vi "Verify Cycle Rounting time.vi"(0 "GEA2 Reference In":refnum<k24>, 5 "ECT Data In":T1, 11 "Error In":errorcluster) -> (4 "GEA2 Reference Out":refnum<k24>, 6 "Routing ECT pass/fail":bool, 8 "Report Text Cycle Routing":string, 15 "Error Out":errorcluster)   [LabVIEW 2016, in "TLMB.lvlib"]
doc: "This vi can be used to read ERD every 1 sec for user selected repeat counts."
uses:
  Projects/TLMB.lvlib
  Q:/Common/DLLs/GEA3/GeaCommunication.dll
  Common/DLLs/GEA3/GeaCommunication.dll
  Controls/ECT.ctl
  Common/LabVIEW GEA2 Toolkit/LabVIEW_GEA2_Toolkit.lvlibp/type defs/Source_Destination.ctl
  Common/LabVIEW GEA2 Toolkit/LabVIEW_GEA2_Toolkit.lvlibp/type defs/ERD Read Data In.ctl
  Common/LabVIEW GEA2 Toolkit/LabVIEW_GEA2_Toolkit.lvlibp/type defs/Data Type.ctl
  Common/LabVIEW GEA2 Toolkit/LabVIEW_GEA2_Toolkit.lvlibp
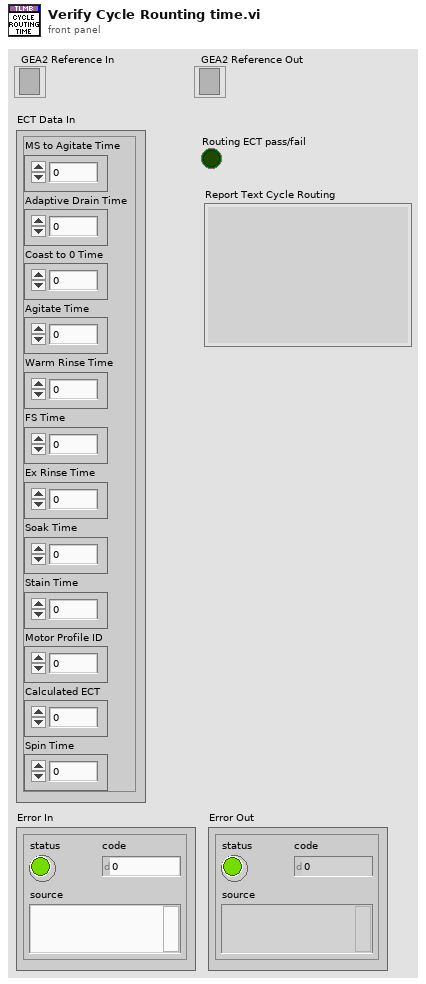
[diagram p1: front panel]
types:
  T1 = typedef "TLMB.lvlib/ECT.ctl" = cluster{"MS to Agitate Time":u16, "Adaptive Drain Time":u16, "Coast to 0 Time":u16, "Agitate Time":u16, "Warm Rinse Time":u16, "FS Time":u16, "Ex Rinse Time":u16, "Soak Time":u16, "Stain Time":u16, "Motor Profile ID":u16, "Calculated ECT":u16, "Spin Time":u16}
  T2 = typedef "LabVIEW_GEA2_Toolkit.lvlibp/Source_Destination.ctl" = cluster{"Source":u8, "Destination":u8}
  T3 = typedef "LabVIEW_GEA2_Toolkit.lvlibp/ERD Read Data In.ctl" = cluster{"ERD Number":u16, "Data Type":T4}
  T4 = typedef "LabVIEW_GEA2_Toolkit.lvlibp/Data Type.ctl" = enum16{"string", "boolean", "uint8_t", "uint16_t", "uint32_t", "uint64_t", "int8_t", "int16_t", "int32_t", "int64_t"}
  T5 = enum16{"EQ (==)", "NE (!=)", "GT (>)", "LT (<)", "GE (>=)", "LE (<=)", "GTLT(> <)", "GELE (>= <=)", "GELT (>= <)", "GTLE (> <=)", "LTGT (< >)", "LEGE (<= >=)", "LEGT (<= >)", "LTGE (< >=)", "No Comparison"}
  T6 = typedef "LabVIEW_GEA2_Toolkit.lvlibp/ERD Read Data Out.ctl" = cluster{"ERD Number":u16, "Data":string}
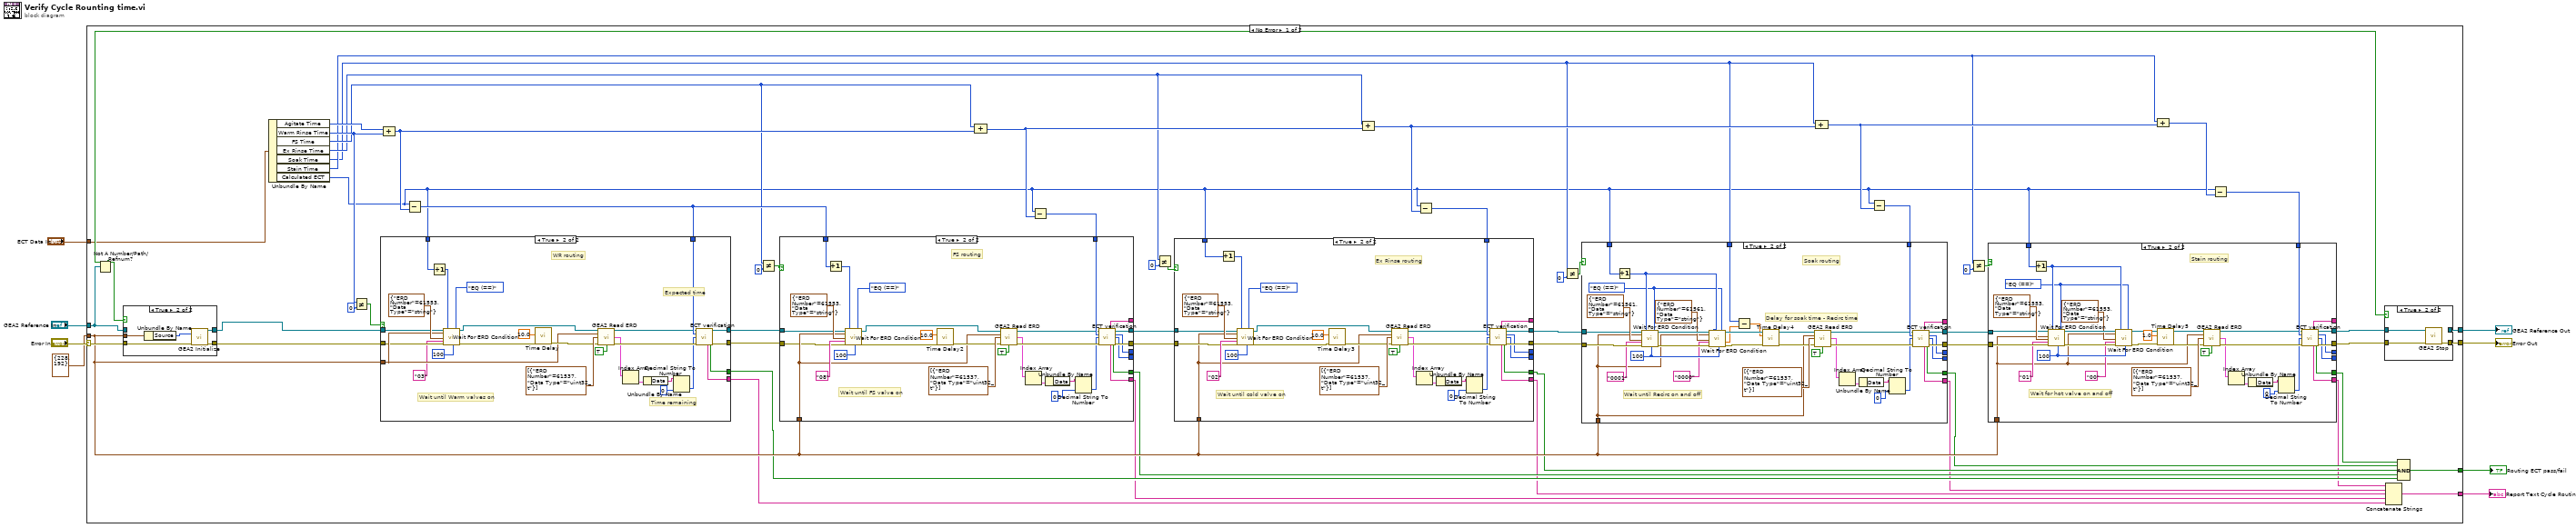
[diagram p0: block diagram]
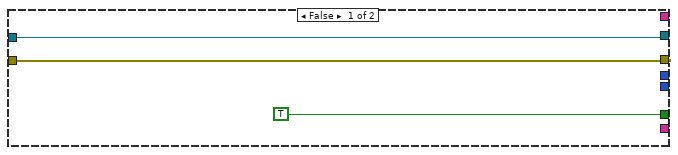
[diagram p2: hidden frame]
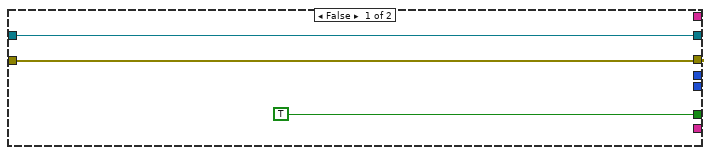
[diagram p3: hidden frame]
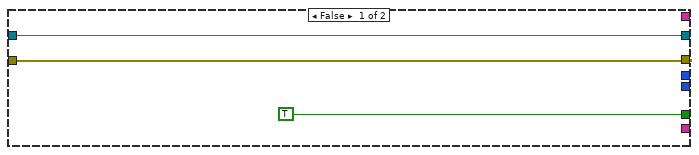
[diagram p4: hidden frame]
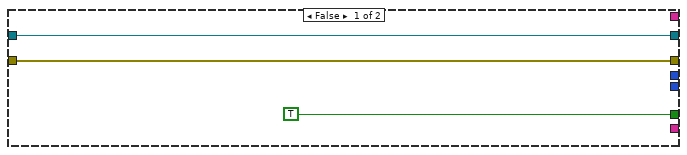
[diagram p5: hidden frame]
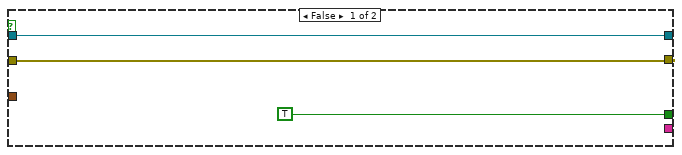
[diagram p6: hidden frame]
diagram:
  n1 = case shown="No Error" "Error In" {
    selector: "Error In" -> [w65 w251]
    tunnel: T2 {"Source"=228, "Destination"=192} ("GEA Inputs") -> [w43 _]
    tunnel: "GEA2 Reference In" -> [w66 w252]
    tunnel: [w62 w252] -> w6
    tunnel: [w64 w251] -> w5
    tunnel: "ECT Data In" -> [w10 _]
    tunnel: [w25 _] -> w3
    tunnel: [w24 _] -> w2
    frame No Error {
      n2 = Not A Number/Path/Refnum?(number/path/refnum=w66) -> (NaN/Path/Refnum?=w63:bool)
      n3 = case shown="True" w63 {
        tunnel: w65 -> [w245 w250]
        tunnel: [w245 w249] -> w9
        tunnel: [w244 w248] -> w12
        tunnel: w43 -> [_ w246]
        tunnel: w66 -> [w244 _]
        frame False {
        }
        frame True {
          n4 = Unbundle By Name(w246) -> ("Source"=w247:u8)
          n5 = call "GEA2 Initialize.vi"("Source Address"=w247, "error in"=w250) -> ("GEA2 Reference Out"=w248:refnum<k24>, "error out"=w249:errorcluster)  [unwired: 11 in, 1 out]
        }
      }
      n6 = Unbundle By Name(w10) -> ("Agitate Time"=w61:u16, "Warm Rinse Time"=w55:u16, "FS Time"=w51:u16, "Ex Rinse Time"=w46:u16, "Soak Time"=w23:u16, "Stain Time"=w36:u16, "Calculated ECT"=w11:u16)
      n7 = Not Equal?(x=w55, y=u16 0) -> (x != y?=w21:bool)
      n8 = Compound Arithmetic op=ADD(w61, w55) -> (w59:u16)
      n9 = Subtract(x=w11, y=w59) -> (x-y=w52:u16)
      n10 = case shown="True" w21 {
        tunnel: [w211 w237] -> w54
        tunnel: [w210 w236] -> w53
        tunnel: w52 -> [_ w230]
        tunnel: [TRUE ("ECT Pass/Fail") w229] -> w35
        tunnel: [_ w228] -> w31
        tunnel: w43 -> [_ w227]
        tunnel: w12 -> [w211 w226]
        tunnel: w9 -> [w210 w225]
        tunnel: w11 -> [_ w215]
        frame False {
        }
        frame True {
          # "Expected time"
          # "Time remaining"
          # "Wait until Warm valves on"
          # "WR routing"
          n11 = Increment(x=w215) -> (x+1=w214:u16)
          n12 = call "Wait For ERD Condition.vi"("GEA2 Reference In"=w226, "GEA Inputs"=w227, "ERD Read Data"=T3 {"ERD Number"=61553, "Data Type"=enum."string"}, "Expected Low"="03", "Error In"=w225, "Timeout (s)"=w214, "Loop Rate (ms)"=u32 100, "Comparison"=T5."EQ (==)") -> ("GEA2 Reference Out"=w217:refnum<k24>, "Error Out"=w216:errorcluster)  [unwired: 7 in, 3 out]
          n13 = call "Time Delay"("error in (no error)"=w216, "Delay Time (s)"=10.0) -> ("error out"=w231:errorcluster)  [unwired: 9 in]
          n14 = call "GEA2 Read ERD.vi"("GEA2 Reference In"=w217, "GEA Inputs"=w227, "Read ERD List"=T3[] [{"ERD Number"=61537, "Data Type"=enum."uint32_t"}], "Error In"=w231, "Verify ERD Response?"=TRUE) -> ("GEA2 Reference Out"=w224:refnum<k24>, "ERD Data Out"=w222:T6[], "Error Out"=w223:errorcluster)  [unwired: 7 in, 1 out]
          n15 = Index Array(array=w222) -> (element=w221:T6)  [unwired: 1 in]
          n16 = Unbundle By Name(w221) -> ("Data"=w220:string)
          n17 = Decimal String To Number(string=w220, default (0L)=u16 0 ("Expected ECT (sec)")) -> (number=w219:u16)  [unwired: 1 in, 1 out]
          n18 = call "ECT verification.vi"(".NET Refnum in"=w224, "Cal ECT (sec)"=w230, "Time remaining (sec)"=w219, "error in"=w223) -> (".NET Refnum out"=w237:refnum<k24>, "ECT Pass/Fail"=w229:bool, "Report Text"=w228:string, "error out"=w236:errorcluster)  [unwired: 5 in, 3 out]
        }
      }
      n19 = Not Equal?(x=w51, y=u16 0) -> (x != y?=w19:bool)
      n20 = Compound Arithmetic op=ADD(w51, w59) -> (w58:u16)
      n21 = Subtract(x=w11, y=w58) -> (x-y=w50:u16)
      n22 = case shown="True" w19 {
        tunnel: [w178 w207] -> w49
        tunnel: [w177 w206] -> w48
        tunnel: w50 -> [_ w200]
        tunnel: [_ w199] -> _
        tunnel: [_ w198] -> _
        tunnel: [_ w197] -> _
        tunnel: [TRUE ("ECT Pass/Fail") w196] -> w34
        tunnel: [_ w195] -> w30
        tunnel: w54 -> [w178 w186]
        tunnel: w53 -> [w177 w185]
        tunnel: w52 -> [_ w182]
        tunnel: w43 -> [_ w187]
        frame False {
        }
        frame True {
          # "Wait until FS valve on"
          # "FS routing"
          n23 = Increment(x=w182) -> (x+1=w181:u16)
          n24 = call "Wait For ERD Condition.vi"("GEA2 Reference In"=w186, "GEA Inputs"=w187, "ERD Read Data"=T3 {"ERD Number"=61553, "Data Type"=enum."string"}, "Expected Low"="08", "Error In"=w185, "Timeout (s)"=w181, "Loop Rate (ms)"=u32 100, "Comparison"=T5."EQ (==)") -> ("GEA2 Reference Out"=w184:refnum<k24>, "Error Out"=w183:errorcluster)  [unwired: 7 in, 3 out]
          n25 = call "Time Delay2"("error in (no error)"=w183, "Delay Time (s)"=10.0) -> ("error out"=w201:errorcluster)  [unwired: 9 in]
          n26 = call "GEA2 Read ERD.vi"("GEA2 Reference In"=w184, "GEA Inputs"=w187, "Read ERD List"=T3[] [{"ERD Number"=61537, "Data Type"=enum."uint32_t"}], "Error In"=w201, "Verify ERD Response?"=TRUE) -> ("GEA2 Reference Out"=w194:refnum<k24>, "ERD Data Out"=w192:T6[], "Error Out"=w193:errorcluster)  [unwired: 7 in, 1 out]
          n27 = Index Array(array=w192) -> (element=w191:T6)  [unwired: 1 in]
          n28 = Unbundle By Name(w191) -> ("Data"=w190:string)
          n29 = Decimal String To Number(string=w190, default (0L)=u16 0 ("Expected ECT (sec)")) -> (number=w189:u16)  [unwired: 1 in, 1 out]
          n30 = call "ECT verification.vi"(".NET Refnum in"=w194, "Cal ECT (sec)"=w200, "Time remaining (sec)"=w189, "error in"=w193) -> ("Expected SSD"=w199:string, ".NET Refnum out"=w207:refnum<k24>, "Expected ECT (sec)"=w198:u16, "Actual ECT (sec)"=w197:u16, "ECT Pass/Fail"=w196:bool, "Report Text"=w195:string, "error out"=w206:errorcluster)  [unwired: 5 in]
        }
      }
      n31 = Not Equal?(x=w46, y=u16 0) -> (x != y?=w17:bool)
      n32 = Compound Arithmetic op=ADD(w46, w58) -> (w57:u16)
      n33 = Subtract(x=w11, y=w57) -> (x-y=w47:u16)
      n34 = case shown="True" w17 {
        tunnel: [w145 w174] -> w38
        tunnel: [w144 w173] -> w37
        tunnel: w47 -> [_ w167]
        tunnel: [_ w166] -> _
        tunnel: [_ w165] -> _
        tunnel: [_ w164] -> _
        tunnel: [TRUE ("ECT Pass/Fail") w163] -> w29
        tunnel: [_ w162] -> w28
        tunnel: w49 -> [w145 w154]
        tunnel: w48 -> [w144 w153]
        tunnel: w11 -> [_ w149]
        tunnel: w43 -> [_ w150]
        frame False {
        }
        frame True {
          # "Wait until cold valve on"
          # "Ex Rinse routing"
          n35 = Increment(x=w149) -> (x+1=w148:u16)
          n36 = call "Wait For ERD Condition.vi"("GEA2 Reference In"=w154, "GEA Inputs"=w150, "ERD Read Data"=T3 {"ERD Number"=61553, "Data Type"=enum."string"}, "Expected Low"="02", "Error In"=w153, "Timeout (s)"=w148, "Loop Rate (ms)"=u32 100, "Comparison"=T5."EQ (==)") -> ("GEA2 Reference Out"=w152:refnum<k24>, "Error Out"=w151:errorcluster)  [unwired: 7 in, 3 out]
          n37 = call "Time Delay3"("error in (no error)"=w151, "Delay Time (s)"=10.0) -> ("error out"=w168:errorcluster)  [unwired: 9 in]
          n38 = call "GEA2 Read ERD.vi"("GEA2 Reference In"=w152, "GEA Inputs"=w150, "Read ERD List"=T3[] [{"ERD Number"=61537, "Data Type"=enum."uint32_t"}], "Error In"=w168, "Verify ERD Response?"=TRUE) -> ("GEA2 Reference Out"=w161:refnum<k24>, "ERD Data Out"=w159:T6[], "Error Out"=w160:errorcluster)  [unwired: 7 in, 1 out]
          n39 = Index Array(array=w159) -> (element=w158:T6)  [unwired: 1 in]
          n40 = Unbundle By Name(w158) -> ("Data"=w157:string)
          n41 = Decimal String To Number(string=w157, default (0L)=u16 0 ("Expected ECT (sec)")) -> (number=w156:u16)  [unwired: 1 in, 1 out]
          n42 = call "ECT verification.vi"(".NET Refnum in"=w161, "Cal ECT (sec)"=w167, "Time remaining (sec)"=w156, "error in"=w160) -> ("Expected SSD"=w166:string, ".NET Refnum out"=w174:refnum<k24>, "Expected ECT (sec)"=w165:u16, "Actual ECT (sec)"=w164:u16, "ECT Pass/Fail"=w163:bool, "Report Text"=w162:string, "error out"=w173:errorcluster)  [unwired: 5 in]
        }
      }
      n43 = Not Equal?(x=w23, y=u16 0) -> (x != y?=w15:bool)
      n44 = Compound Arithmetic op=ADD(w23, w57) -> (w56:u16)
      n45 = Subtract(x=w11, y=w56) -> (x-y=w45:u16)
      n46 = case shown="True" w15 {
        tunnel: [w106 w141] -> w41
        tunnel: [w105 w140] -> w42
        tunnel: w45 -> [_ w130]
        tunnel: [_ w129] -> _
        tunnel: [_ w128] -> _
        tunnel: [_ w127] -> _
        tunnel: [TRUE ("ECT Pass/Fail") w126] -> w33
        tunnel: [_ w125] -> w27
        tunnel: w38 -> [w106 w124]
        tunnel: w37 -> [w105 w123]
        tunnel: w11 -> [_ w110]
        tunnel: w43 -> [_ w114]
        tunnel: w23 -> [_ w113]
        frame False {
        }
        frame True {
          w107 = T5."EQ (==)" ("Comparison")
          w135 = u32 100 ("Loop Rate (ms)")
          # "Delay for soak time - Recirc time"
          # "Wait until Recirc on and off"
          # "Soak routing"
          n47 = Increment(x=w110) -> (x+1=w109:u16)
          n48 = call "Wait For ERD Condition.vi"("GEA2 Reference In"=w124, "GEA Inputs"=w114, "ERD Read Data"=T3 {"ERD Number"=61561, "Data Type"=enum."string"}, "Expected Low"="0001", "Error In"=w123, "Timeout (s)"=w109, "Loop Rate (ms)"=w135, "Comparison"=w107) -> ("GEA2 Reference Out"=w138:refnum<k24>, "Error Out"=w137:errorcluster)  [unwired: 7 in, 3 out]
          n49 = call "Wait For ERD Condition.vi"("GEA2 Reference In"=w138, "GEA Inputs"=w114, "ERD Read Data"=T3 {"ERD Number"=61561, "Data Type"=enum."string"}, "Expected Low"="0000", "Error In"=w137, "Timeout (s)"=w109, "Loop Rate (ms)"=w135, "Comparison"=w107) -> ("GEA2 Reference Out"=w136:refnum<k24>, "Execution Time"=w112:dbl, "Error Out"=w132:errorcluster)  [unwired: 7 in, 2 out]
          n50 = Subtract(x=w113, y=w112) -> (x-y=w111:dbl)
          n51 = call "Time Delay4"("error in (no error)"=w132, "Delay Time (s)"=w111) -> ("error out"=w131:errorcluster)  [unwired: 9 in]
          n52 = call "GEA2 Read ERD.vi"("GEA2 Reference In"=w136, "GEA Inputs"=w114, "Read ERD List"=T3[] [{"ERD Number"=61537, "Data Type"=enum."uint32_t"}], "Error In"=w131, "Verify ERD Response?"=TRUE) -> ("GEA2 Reference Out"=w122:refnum<k24>, "ERD Data Out"=w120:T6[], "Error Out"=w121:errorcluster)  [unwired: 7 in, 1 out]
          n53 = Index Array(array=w120) -> (element=w119:T6)  [unwired: 1 in]
          n54 = Unbundle By Name(w119) -> ("Data"=w118:string)
          n55 = Decimal String To Number(string=w118, default (0L)=u16 0 ("Expected ECT (sec)")) -> (number=w117:u16)  [unwired: 1 in, 1 out]
          n56 = call "ECT verification.vi"(".NET Refnum in"=w122, "Cal ECT (sec)"=w130, "Time remaining (sec)"=w117, "error in"=w121) -> ("Expected SSD"=w129:string, ".NET Refnum out"=w141:refnum<k24>, "Expected ECT (sec)"=w128:u16, "Actual ECT (sec)"=w127:u16, "ECT Pass/Fail"=w126:bool, "Report Text"=w125:string, "error out"=w140:errorcluster)  [unwired: 5 in]
        }
      }
      n57 = Not Equal?(x=w36, y=u16 0) -> (x != y?=w13:bool)
      n58 = Compound Arithmetic op=ADD(w36, w56) -> (w60:u16)
      n59 = Subtract(x=w11, y=w60) -> (x-y=w44:u16)
      n60 = case shown="True" w13 {
        tunnel: [w67 w102] -> w40
        tunnel: [w69 w101] -> w39
        tunnel: w44 -> [_ w91]
        tunnel: [_ w90] -> _
        tunnel: [_ w89] -> _
        tunnel: [_ w88] -> _
        tunnel: [TRUE ("ECT Pass/Fail") w87] -> w32
        tunnel: [_ w86] -> w26
        tunnel: w42 -> [w69 w85]
        tunnel: w11 -> [_ w74]
        tunnel: w43 -> [_ w76]
        tunnel: w41 -> [w67 w75]
        frame False {
        }
        frame True {
          w70 = T5."EQ (==)" ("Comparison")
          w96 = u32 100 ("Loop Rate (ms)")
          # "Wait for hot valve on and off"
          # "Stain routing"
          n61 = Increment(x=w74) -> (x+1=w73:u16)
          n62 = call "Wait For ERD Condition.vi"("GEA2 Reference In"=w75, "GEA Inputs"=w76, "ERD Read Data"=T3 {"ERD Number"=61553, "Data Type"=enum."string"}, "Expected Low"="01", "Error In"=w85, "Timeout (s)"=w73, "Loop Rate (ms)"=w96, "Comparison"=w70) -> ("GEA2 Reference Out"=w99:refnum<k24>, "Error Out"=w98:errorcluster)  [unwired: 7 in, 3 out]
          n63 = call "Wait For ERD Condition.vi"("GEA2 Reference In"=w99, "GEA Inputs"=w76, "ERD Read Data"=T3 {"ERD Number"=61553, "Data Type"=enum."string"}, "Expected Low"="00", "Error In"=w98, "Timeout (s)"=w73, "Loop Rate (ms)"=w96, "Comparison"=w70) -> ("GEA2 Reference Out"=w97:refnum<k24>, "Error Out"=w93:errorcluster)  [unwired: 7 in, 3 out]
          n64 = call "Time Delay5"("error in (no error)"=w93, "Delay Time (s)"=1.0) -> ("error out"=w92:errorcluster)  [unwired: 9 in]
          n65 = call "GEA2 Read ERD.vi"("GEA2 Reference In"=w97, "GEA Inputs"=w76, "Read ERD List"=T3[] [{"ERD Number"=61537, "Data Type"=enum."uint32_t"}], "Error In"=w92, "Verify ERD Response?"=TRUE) -> ("GEA2 Reference Out"=w84:refnum<k24>, "ERD Data Out"=w82:T6[], "Error Out"=w83:errorcluster)  [unwired: 7 in, 1 out]
          n66 = Index Array(array=w82) -> (element=w81:T6)  [unwired: 1 in]
          n67 = Unbundle By Name(w81) -> ("Data"=w80:string)
          n68 = Decimal String To Number(string=w80, default (0L)=u16 0 ("Expected ECT (sec)")) -> (number=w79:u16)  [unwired: 1 in, 1 out]
          n69 = call "ECT verification.vi"(".NET Refnum in"=w84, "Cal ECT (sec)"=w91, "Time remaining (sec)"=w79, "error in"=w83) -> ("Expected SSD"=w90:string, ".NET Refnum out"=w102:refnum<k24>, "Expected ECT (sec)"=w89:u16, "Actual ECT (sec)"=w88:u16, "ECT Pass/Fail"=w87:bool, "Report Text"=w86:string, "error out"=w101:errorcluster)  [unwired: 5 in]
        }
      }
      n70 = case shown="True" w63 {
        tunnel: [w240 w243] -> w64
        tunnel: w40 -> [w239 w242]
        tunnel: w39 -> [w240 w241]
        tunnel: [w239 _] -> w62
        frame False {
        }
        frame True {
          n71 = call "GEA2 Stop.vi"("GEA2 Reference In"=w242, "Error In"=w241) -> ("Error Out"=w243:errorcluster)  [unwired: 13 in]
        }
      }
      n72 = Concatenate Strings(w26, w27, w28, w30, w31) -> (w24:string)
      n73 = Compound Arithmetic op=AND(w32, w33, w29, w34, w35) -> (w25:bool)
    }
    frame Error {
    }
  }
  "GEA2 Reference Out" <- w6
  "Error Out" <- w5
  "Routing ECT pass/fail" <- w3
  "Report Text Cycle Routing" <- w2
